vi "Get Timeout.vi"(8 "error in (no error)":errorcluster, 11 "SwipeMenu in":refnum<class "SwipeMenu.lvclass">) -> (0 "error out":errorcluster, 2 "Timeout":i32, 3 "SwipeMenu out":refnum<class "SwipeMenu.lvclass">)   [LabVIEW 2019, in "SwipeMenu.lvclass"]
uses:
  SwipeMenu.lvclass
  SwipeMenu.lvclass/SwipeMenu.ctl
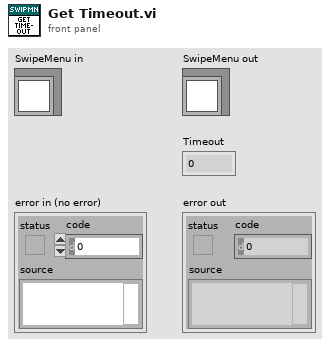
[diagram p1: front panel]
types:
  T1 = typedef "SwipeMenu.lvclass/State Data.ctl" = cluster{"State":enum16{"Idle", "Mouse Nav", "Slowdown", "Button Nav"}, "Timeout":i32, "Time":timestamp, "Position":i32, "Scroll Position":i16, "Rate":dbl, "Direction":enum16{"Left", "Right"}}
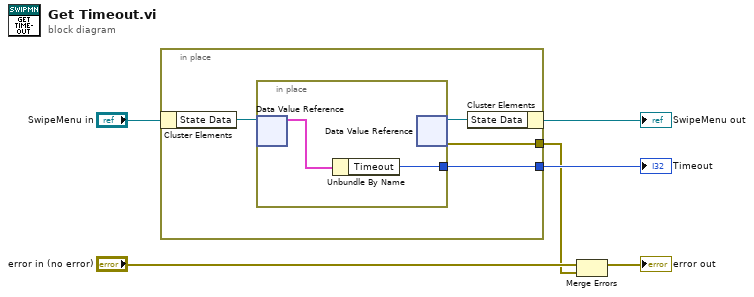
[diagram p0: block diagram]
diagram:
  n1 = in-place {
    in-place-border: [w8] -> w4
    in-place-border: [w7] -> w1
    n2 = in-place-cluster #1("SwipeMenu in") -> ("State Data"=w10:refnum<data-value>)
    n3 = in-place {
      in-place-border: [w11] -> w8
      n4 = in-place-dvr #2(w10) -> (w12:T1)  [unwired: 1 out]
      n5 = Unbundle By Name(w12) -> ("Timeout"=w11:i32)
      n6 = in-place-dvr #2() -> (w9:refnum<data-value>, w7:errorcluster)  [unwired: 1 in]
    }
    n7 = in-place-cluster #1("State Data"=w9) -> (→"SwipeMenu out":refnum<class "SwipeMenu.lvclass">)
  }
  "Timeout" <- w4
  n8 = Merge Errors("error in (no error)", w1) -> (→"error out":errorcluster)
